vi "__Alicat SD_Hardware_Module_v2.vi"(5 "Used ?":bool=TRUE, 7 "Command":T2, 8 "error in (no error)":errorcluster, 9 "SetPoint (64000=FullScale)":i32=32000 min=0 max=64000 step=1, 10 "Address":string="A", 11 "VISA resource name":refnum<visa-resource-name>="COM6") -> (0 "error out":errorcluster, 1 "ParsedReading":T1={"ID"="", "Pressure"=13.55, "Temperature"=28.56, "Volumetric"=-1.9, "Mass"=-1.7, "SetPoint"=250.0, "Gas"="", "Total"=250.0} {"Total" format="%.2f"; "SetPoint" format="%.2f"; "Mass" format="%.2f"; "Volumetric" format="%.2f"; "Temperature" format="%.2f"; "Pressure" format="%.2f"}, 2 "AlicatResponse":string="A +013.53 +023.20 +0000.0 +0000.0 0250.0     Air\r", 3 "Timeout":bool)   [LabVIEW 2017]
uses:
  __Alicat SD_Hardware_Module.ctl
  __Alicat SD_ReadingCluster.ctl
  <vilib>/Instr/_visa.llb/VISA Configure Serial Port (Instr).vi
panel:
  out "Bytes":u32
  in  "Timeout(s)":dbl=2.0
  # "Input Data"
  # "Output Data"
  # "ID  P(PSIA) TEMP(C) FLOW(vol) FLOW(mass)  SP TOTAL  GAS"
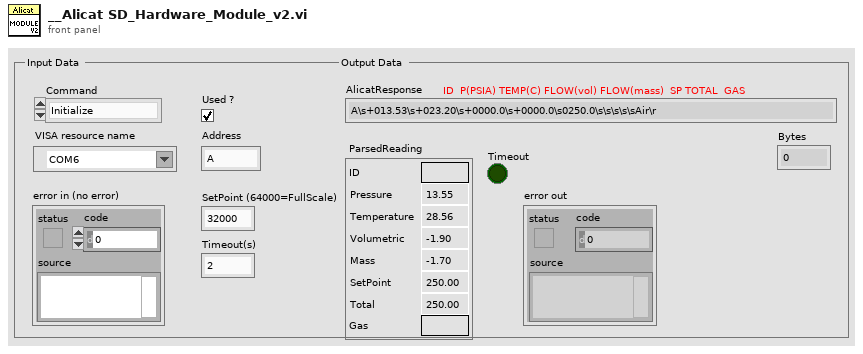
[diagram p1: front panel]
types:
  T1 = typedef "__Alicat SD_ReadingCluster.ctl" = cluster{"ID":string, "Pressure":sgl, "Temperature":sgl, "Volumetric":sgl, "Mass":sgl, "SetPoint":sgl, "Gas":string, "Total":sgl}
  T2 = typedef "__Alicat SD_Hardware_Module.ctl" = enum16{"Initialize", "Send Setpoint", "Read Data", "Change Address", "Shutdown"}
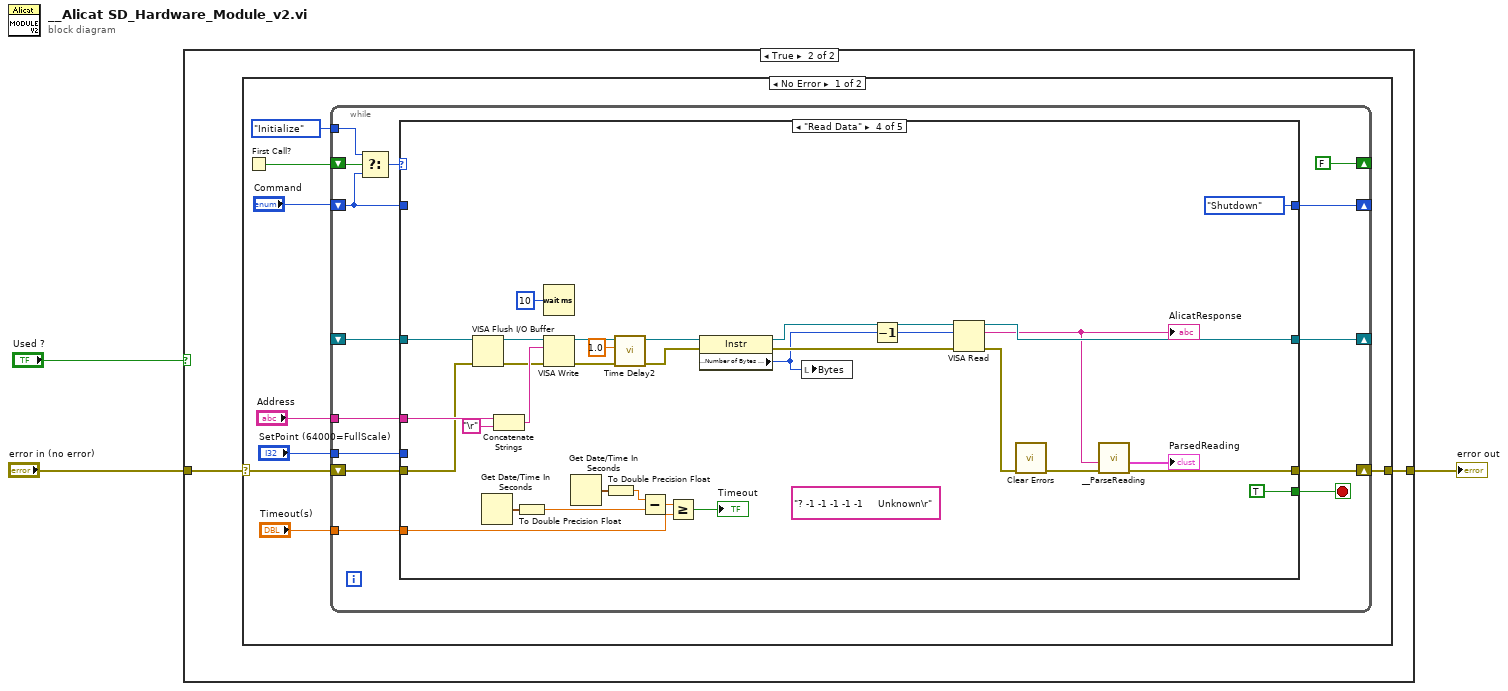
[diagram p0: block diagram]
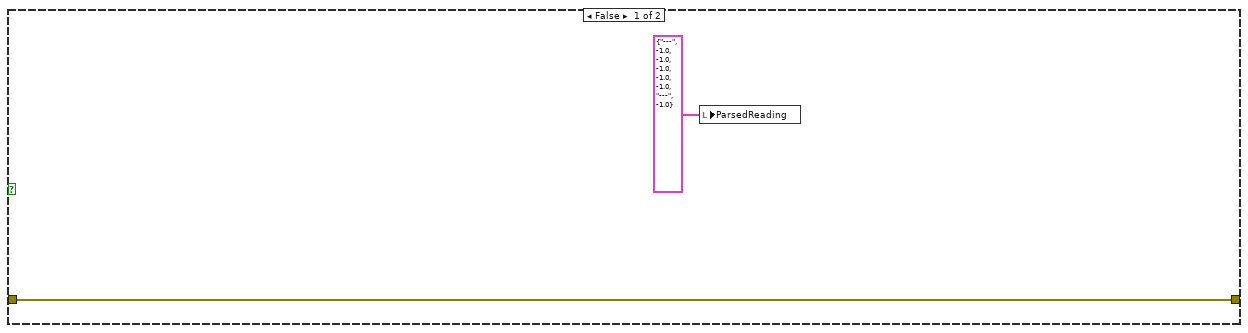
[diagram p2: hidden frame]
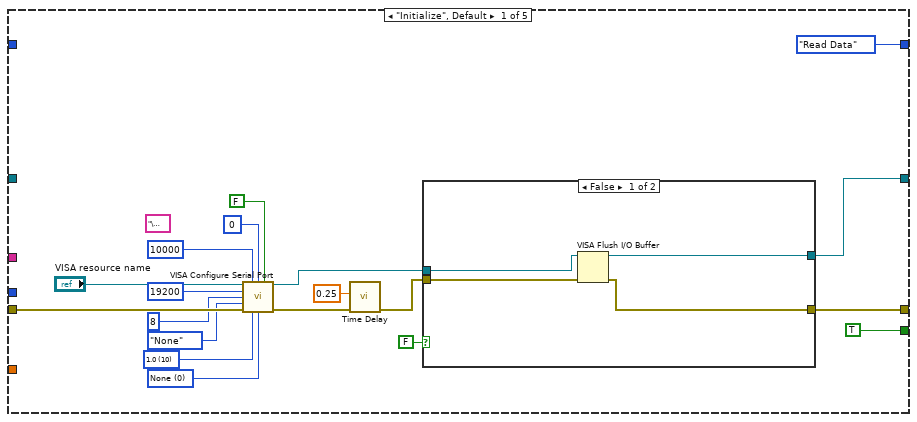
[diagram p3: hidden frame]
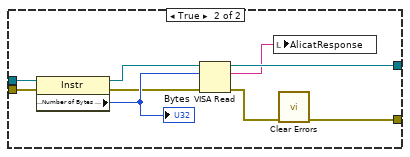
[diagram p4: hidden frame]
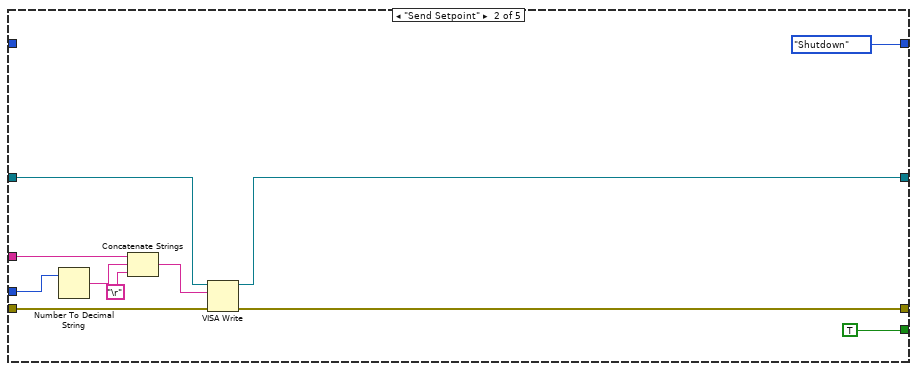
[diagram p5: hidden frame]
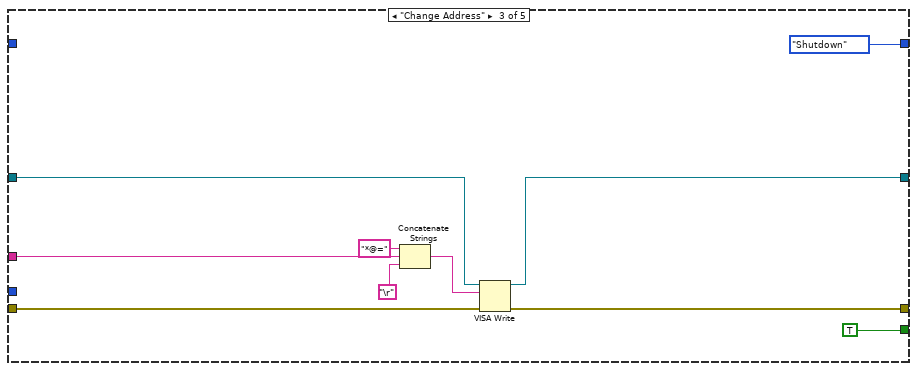
[diagram p6: hidden frame]
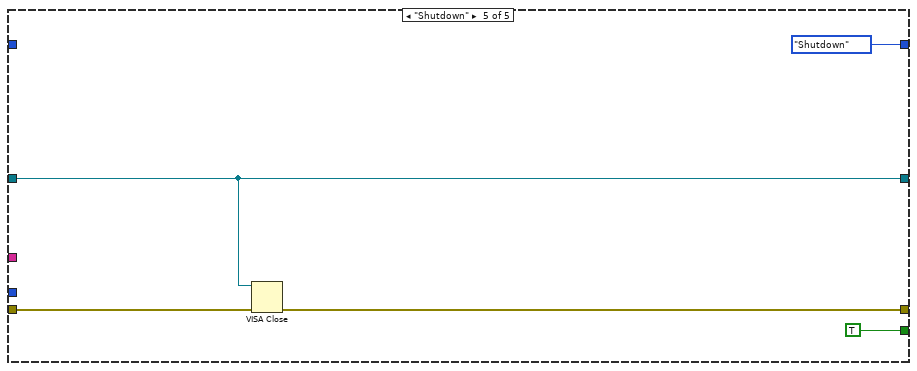
[diagram p7: hidden frame]
diagram:
  n1 = case shown="True" "Used ?" {
    tunnel: "error in (no error)" -> [w5 w7]
    tunnel: [w5 w6] -> w2
    frame False {
      n2 = local write "ParsedReading"(T1 {"ID"="---", "Pressure"=-1.0, "Temperature"=-1.0, "Volumetric"=-1.0, "Mass"=-1.0, "SetPoint"=-1.0, "Gas"="---", "Total"=-1.0} ("ParsedReading")) -> ()
    }
    frame True {
      n3 = case shown="No Error" w7 {
        selector: w7 -> [w13 w119]
        tunnel: [w12 w119] -> w6
        frame No Error {
          n4 = First Call?() -> (First Call?: T/F=w15:bool)
          n5 = while {
            shift-right: [w21] -> _
            shift-left: "Command" -> [w22]
            shift-right: [w24] -> w12
            shift-left: w13 -> [w25]
            shift-right: [FALSE ("First Call?: T/F")] -> _
            shift-left: w15 -> [w29]
            tunnel: __Alicat_SD_Hardware_Module."Initialize" ("t") -> [w28]
            shift-right: [w19] -> _
            shift-left: _ -> [w20]
            tunnel: "Address" -> [w18]
            tunnel: "SetPoint (64000=FullScale)" -> [w17]
            tunnel: "Timeout(s)" -> [w16]
            stop <- w26 stop-if-true
            n6 = Select(t=w28, s=w29, f=w22) -> (s? t:f=w27:T2)
            n7 = case shown="\"Read Data\"" w27 {
              tunnel: [TRUE TRUE TRUE TRUE TRUE] -> w26
              tunnel: w25 -> [w45 w70 w80 w87 w116]
              tunnel: [w37 w69 w79 w88 w115] -> w24
              tunnel: w22 -> [_ _ _ _ _]
              tunnel: [__Alicat_SD_Hardware_Module."Read Data" ("t") __Alicat_SD_Hardware_Module."Shutdown" ("t") __Alicat_SD_Hardware_Module."Shutdown" ("t") __Alicat_SD_Hardware_Module."Shutdown" ("t") __Alicat_SD_Hardware_Module."Shutdown" ("t")] -> w21
              tunnel: w20 -> [_ w65 w76 w85 w114]
              tunnel: [w39 w64 w75 w108 w114] -> w19
              tunnel: w18 -> [_ w68 w78 w104 _]
              tunnel: w17 -> [_ w63 _ _ _]
              tunnel: w16 -> [_ _ _ w109 _]
              frame "Initialize", Default {
                (unwired) "\u0000"
                w32 = u16 0 items=["None", "XON/XOFF", "RTS/CTS", "XON/XOFF & RTS/CTS", "DTR/DSR", "XON/XOFF & DTR/DSR"] ("flow control (0:none)")
                w33 = u16 10 items=["1.0"=10, "1.5"=15, "2.0"=20] ("stop bits (10: 1 bit)")
                n8 = call-poly "VISA Configure Serial Port"("VISA resource name"="VISA resource name", "timeout (10sec)"=u32 10000, "termination char\n(0xA = '\\n' = LF)"=u8 0 ("termination char\n(0xA = '\\n' = LF)"), "Enable Termination\nChar (T)"=FALSE ("Enable Termination\nChar (T)"), "baud rate (9600)"=u32 19200, "data bits (8)"=u16 8, "parity (0:none)"=enum16{"None", "Odd", "Even", "Mark", "Space"}."None", "error in (no error)"=w45, "stop bits (10: 1 bit)"=w33, "flow control (0:none)"=w32) -> ("VISA resource name out"=w41:refnum<visa-resource-name>, "error out"=w42:errorcluster)  [unwired: 4 in]
                n9 = call "Time Delay"("error in (no error)"=w42, "Delay Time (s)"=0.25) -> ("error out"=w40:errorcluster)  [unwired: 9 in]
                n10 = case shown="False" FALSE {
                  tunnel: w41 -> [w52 w61]
                  tunnel: w40 -> [w49 w60]
                  tunnel: [w51 w59] -> w39
                  tunnel: [w50 w54] -> w37
                  frame False {
                    n11 = VISA Flush I/O Buffer(VISA resource name=w52, error in (no error)=w49) -> (VISA resource name out=w51:refnum<visa-resource-name>, error out=w50:errorcluster)  [unwired: 1 in]
                  }
                  frame True {
                    n12 = property class="Instr"(reference=w61, error in=w60) -> (reference out=w58:refnum<visa-resource-name>, error out=w56:errorcluster, "Serial Settings:Number of Bytes at Serial Port"=w57:u32)
                    "Bytes" <- w57
                    n13 = VISA Read(VISA resource name=w58, byte count=w57, error in (no error)=w56) -> (VISA resource name out=w59:refnum<visa-resource-name>, read buffer=w53:string, error out=w55:errorcluster)  [unwired: 1 out]
                    n14 = local write "AlicatResponse"(w53) -> ()
                    n15 = call <vilib>:"Clear Errors.vi"("error in (no error)"=w55) -> ("error out"=w54:errorcluster)  [unwired: 5 in, 1 out]
                  }
                }
              }
              frame "Send Setpoint" {
                n16 = Number To Decimal String(number=w63) -> (decimal integer string=w67:string)  [unwired: 1 in]
                n17 = Concatenate Strings(w68, w67, "\r") -> (w66:string)
                n18 = VISA Write(VISA resource name=w65, write buffer=w66, error in (no error)=w70) -> (VISA resource name out=w64:refnum<visa-resource-name>, error out=w69:errorcluster)  [unwired: 1 out]
              }
              frame "Change Address" {
                n19 = Concatenate Strings("*@=" ("string"), w78, "\r") -> (w77:string)
                n20 = VISA Write(VISA resource name=w76, write buffer=w77, error in (no error)=w80) -> (VISA resource name out=w75:refnum<visa-resource-name>, error out=w79:errorcluster)  [unwired: 1 out]
              }
              frame "Read Data" {
                (unwired) "? -1 -1 -1 -1 -1     Unknown\r" ("AlicatResponse")
                n21 = VISA Flush I/O Buffer(VISA resource name=w85, error in (no error)=w87) -> (VISA resource name out=w84:refnum<visa-resource-name>, error out=w86:errorcluster)  [unwired: 1 in]
                n22 = Get Date/Time In Seconds() -> (seconds since 1Jan1904=w110:timestamp)
                n23 = Concatenate Strings(w104, "\r") -> (w107:string)
                n24 = To Double Precision Float(number=w110) -> (double precision float=w111:dbl)
                n25 = Wait (ms)(milliseconds to wait=u32 10) -> ()  [unwired: 1 out]
                n26 = VISA Write(VISA resource name=w84, write buffer=w107, error in (no error)=w86) -> (VISA resource name out=w105:refnum<visa-resource-name>, error out=w93:errorcluster)  [unwired: 1 out]
                n27 = Get Date/Time In Seconds() -> (seconds since 1Jan1904=w99:timestamp)
                n28 = To Double Precision Float(number=w99) -> (double precision float=w98:dbl)
                n29 = call "Time Delay2"("error in (no error)"=w93, "Delay Time (s)"=1.0) -> ("error out"=w92:errorcluster)  [unwired: 9 in]
                n30 = Subtract(x=w98, y=w111) -> (x-y=w97:dbl)
                n31 = Greater Or Equal?(x=w97, y=w109) -> (x >= y?=→"Timeout":bool)
                n32 = property class="Instr"(reference=w105, error in=w92) -> (reference out=w94:refnum<visa-resource-name>, error out=w95:errorcluster, "Serial Settings:Number of Bytes at Serial Port"=w91:u32)
                n33 = local write "Bytes"(w91) -> ()
                n34 = Decrement(x=w91) -> (x-1=w83:u32)
                n35 = VISA Read(VISA resource name=w94, byte count=w83, error in (no error)=w95) -> (VISA resource name out=w108:refnum<visa-resource-name>, read buffer=w102:string, error out=w90:errorcluster)  [unwired: 1 out]
                "AlicatResponse" <- w102
                n36 = call <vilib>:"Clear Errors.vi"("error in (no error)"=w90) -> ("error out"=w89:errorcluster)  [unwired: 5 in, 1 out]
                n37 = call "__ParseReading.vi"("error in (no error)"=w89, "AlicatResponse"=w102) -> ("error out"=w88:errorcluster, "ParsedReading"=→"ParsedReading":T1)  [unwired: 8 in]
              }
              frame "Shutdown" {
                n38 = VISA Close(VISA resource name=w114, error in (no error)=w116) -> (error out=w115:errorcluster)
              }
            }
          }
        }
        frame Error {
        }
      }
    }
  }
  "error out" <- w2
